vi "Create.vi"(4 "Actor Ref":refnum<vi>, 5 "Queue of Error":refnum<queue>, 6 "Creator Attributes":refnum<class "Attributes.lvclass">, 7 "Alias":string, 9 "Queue of Self Attributes":refnum<queue>, 10 "Actor in":refnum<class "Actor.lvclass">) -> (0 "Error out":errorcluster, 1 "Event Ref":refnum<event-registration>, 2 "Actor out":refnum<class "Actor.lvclass">)   [LabVIEW 2025, in "jettl.lvlib" / "Actor.lvlib"]
uses:
  Actor.lvlib
  Actor/Actor.lvclass
  Attributes/Attributes/Attributes.lvclass
  Msg/Msg.lvclass
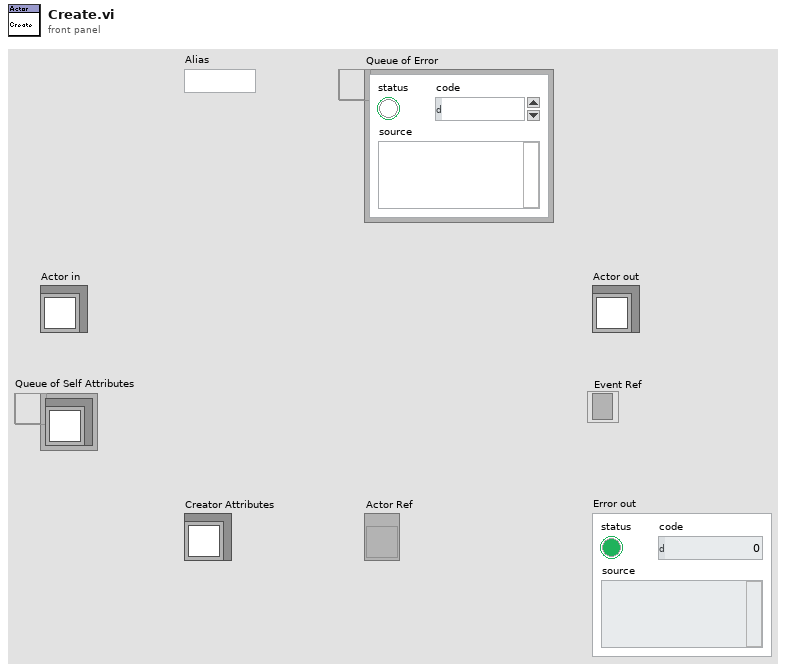
[diagram p1: front panel]
types:
  T1 = typedef "jettl.lvlib/Actor.lvlib/Msg Set.ctl" = set{refnum<class "Msg.lvclass">}
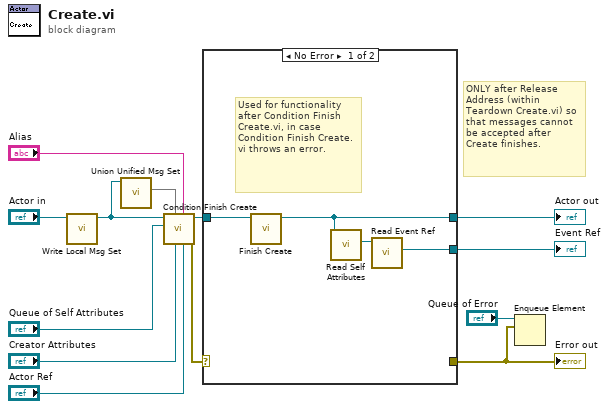
[diagram p0: block diagram]
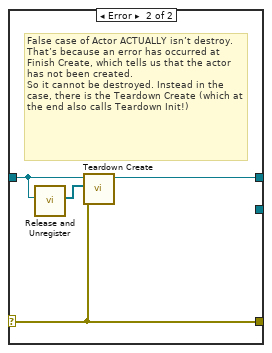
[diagram p2: hidden frame]
diagram:
  # "ONLY after Release Address (within Teardown Create.vi) so that messages cannot be accepted after Create finishes."
  n1 = call-dynamic "Write Local Msg Set.vi"("Actor in"="Actor in") -> ("Actor out"=w7:refnum<class "Actor.lvclass">)  [unwired: 10 in]
  n2 = call-dynamic "Union Unified Msg Set.vi"("Get Actor in"=w7) -> ("Unified Msg Set"=w13:T1)  [unwired: 10 in]
  n3 = call-dynamic "Condition Finish Create.vi"("Actor Ref"="Actor Ref", "Alias"="Alias", "Creator Attributes"="Creator Attributes", "Unified Msg Set"=w13, "Queue of Self Attributes"="Queue of Self Attributes", "Actor in"=w7) -> ("Error out"=w3:errorcluster, "Actor out"=w6:refnum<class "Actor.lvclass">)  [unwired: 4 in]
  n4 = case shown="No Error" w3 {
    selector: w3 -> [_ w18]
    tunnel: w6 -> [w15 w21]
    tunnel: [w16 _] -> w1
    tunnel: [_ w18] -> w4
    tunnel: [w14 w19] -> w5
    frame No Error {
      # "Used for functionality after Condition Finish Create.vi, in case Condition Finish Create.vi throws an error."
      n5 = call-dynamic "Finish Create.vi"("Actor in"=w15) -> ("Actor out"=w14:refnum<class "Actor.lvclass">)  [unwired: 10 in]
      n6 = call-dynamic "Read Self Attributes.vi"("Actor in"=w14) -> ("Self Attributes"=w17:refnum<class "Attributes.lvclass">)  [unwired: 10 in]
      n7 = call-dynamic "Read Event Ref.vi"("Attributes in"=w17) -> ("Event Ref"=w16:refnum<event-registration>)  [unwired: 10 in]
    }
    frame Error {
      # "False case of Actor ACTUALLY isn’t destroy.\nThat’s because an error has occurred at Finish Create, which tells us that the actor has not been created.\nSo it cannot be destroyed. Instead in the case, there is the Teardown Create (which at the end also calls Teardown Init!)"
      n8 = call "Release and Unregister.vi"("Actor"=w21) -> ("Unhandled Msgs"=w20:refnum<class "Msg.lvclass">[])  [unwired: 10 in]
      n9 = call-dynamic "Teardown Create.vi"("Error in"=w18, "Unhandled Msgs"=w20, "Actor in"=w21) -> ("Actor out"=w19:refnum<class "Actor.lvclass">)  [unwired: 8 in]
    }
  }
  "Actor out" <- w5
  "Error out" <- w4
  "Event Ref" <- w1
  n10 = Enqueue Element(queue="Queue of Error", element=w4) -> ()  [unwired: 2 in, 3 out]
